vi "scan_waveform_yMirrored.vi"(6 "nlines":i32, 8 "flyback":i32, 9 "xpixels":i32, 10 "maxV":dbl, 11 "minV":dbl) -> (2 "xy scan waveform":dbl[][](array[numeric]))   [LabVIEW 2010]
panel:
  out "x waveform":dbl[](graph)
  out "y waveform":dbl[](graph)
  out "ystepSize":dbl
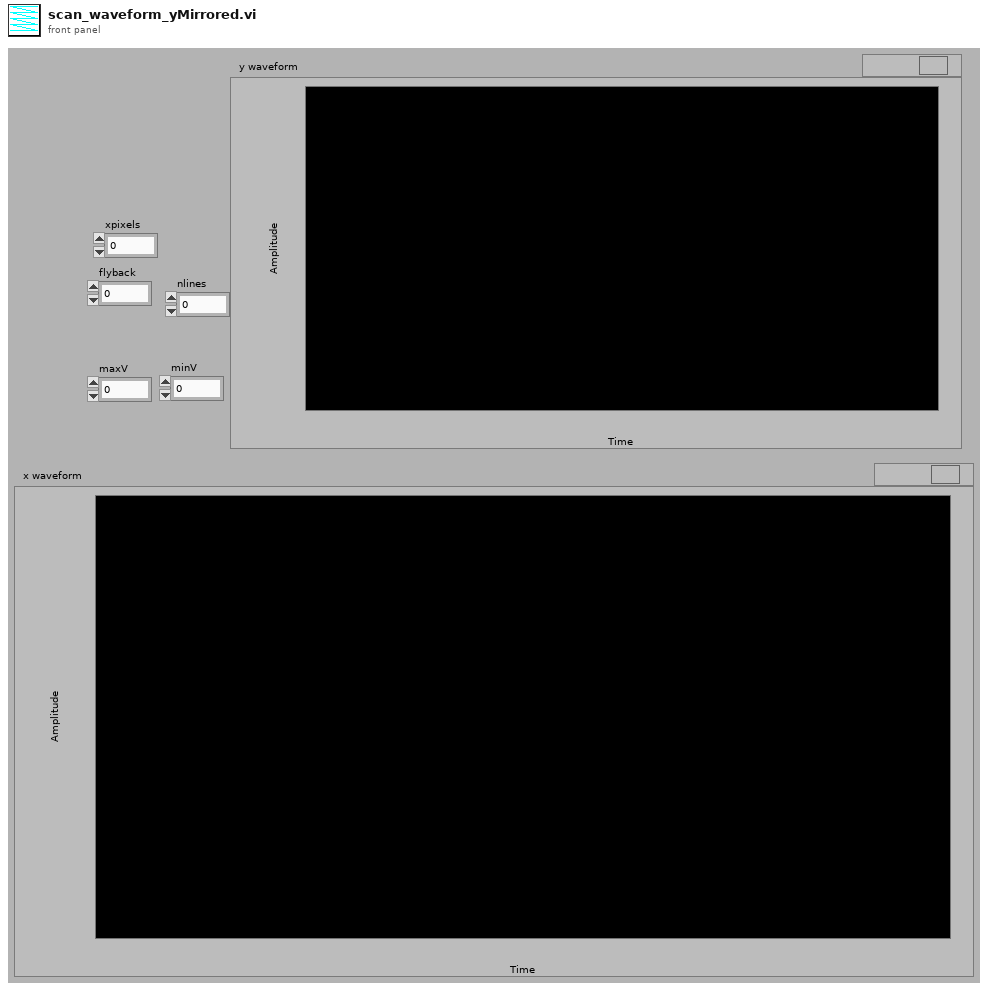
[diagram p1: front panel]
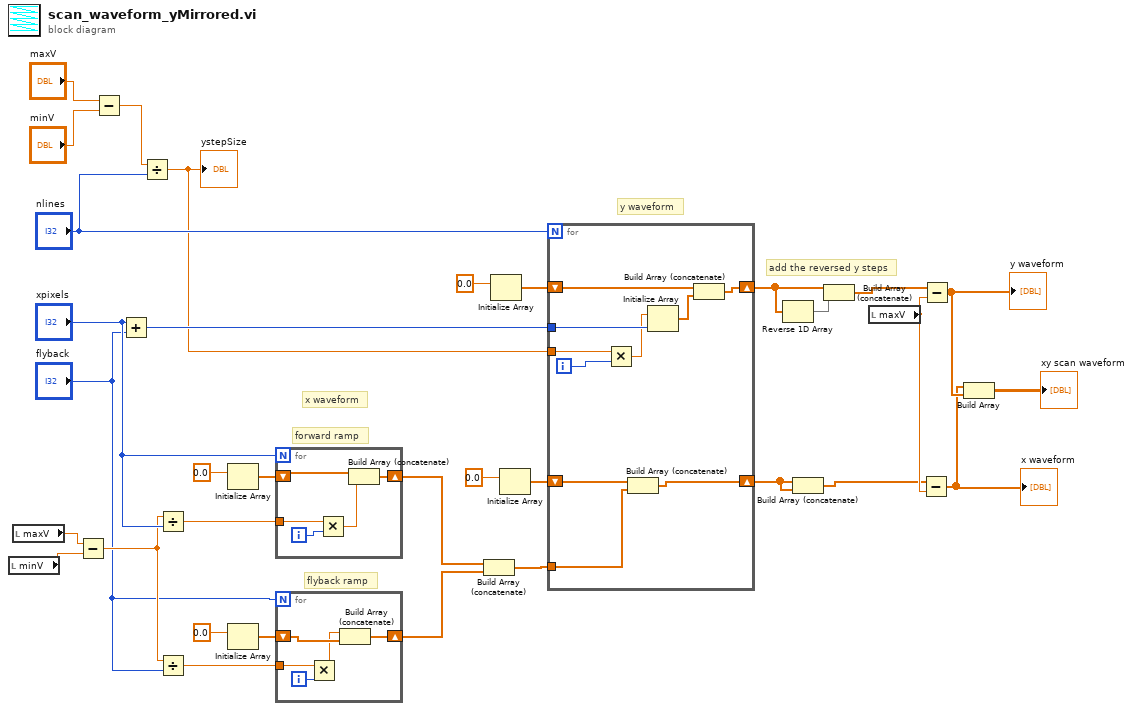
[diagram p0: block diagram]
diagram:
  # "add the reversed y steps"
  # "y waveform"
  # "x waveform"
  # "flyback ramp"
  # "forward ramp"
  n1 = local read "minV"() -> (w24:dbl)
  n2 = local read "maxV"() -> (w25:dbl)
  n3 = Subtract(x=w25, y=w24) -> (x-y=w13:dbl)
  n4 = Subtract(x="maxV", y="minV") -> (x-y=w7:dbl)
  n5 = Add(x="xpixels", y="flyback") -> (x+y=w28:i32)
  n6 = Divide(x=w7, y="nlines") -> (x/y=w10:dbl)
  "ystepSize" <- w10
  n7 = Divide(x=w13, y="xpixels") -> (x/y=w21:dbl)
  n8 = Divide(x=w13, y="flyback") -> (x/y=w20:dbl)
  n9 = Initialize Array(0.0 ("element")) -> (w26:dbl[])  [unwired: 1 out]
  n10 = Initialize Array(0.0 ("element")) -> (w23:dbl[])  [unwired: 1 out]
  n11 = for {
    N: "xpixels" -> [_]
    tunnel: w21 -> [w36]
    shift-right: [w34] -> w19
    shift-left: w26 -> [w38]
    i -> [w37]
    n12 = Multiply(x=w36, y=w37) -> (x*y=w35:dbl)
    n13 = Build Array (concatenate)(w38, w35) -> (w34:dbl[])
  }
  n14 = for {
    N: "flyback" -> [_]
    tunnel: w20 -> [w43]
    shift-right: [w41] -> w11
    shift-left: w23 -> [w40]
    i -> [w42]
    n15 = Multiply(x=w43, y=w42) -> (x*y=w39:dbl)
    n16 = Build Array (concatenate)(w39, w40) -> (w41:dbl[])
  }
  n17 = Build Array (concatenate)(w19, w11) -> (w16:dbl[])
  n18 = Initialize Array(0.0 ("element")) -> (w33:dbl[])  [unwired: 1 out]
  n19 = Initialize Array(0.0 ("element")) -> (w17:dbl[])  [unwired: 1 out]
  n20 = for {
    N: "nlines" -> [_]
    tunnel: w10 -> [w51]
    tunnel: w28 -> [w53]
    shift-right: [w47] -> w2
    shift-left: w33 -> [w48]
    shift-right: [w44] -> w1
    shift-left: w17 -> [w45]
    tunnel: w16 -> [w46]
    i -> [w52]
    n21 = Multiply(x=w51, y=w52) -> (x*y=w50:dbl)
    n22 = Build Array (concatenate)(w45, w46) -> (w44:dbl[])
    n23 = Initialize Array(w50, w53) -> (w49:dbl[])
    n24 = Build Array (concatenate)(w48, w49) -> (w47:dbl[])
  }
  n25 = Reverse 1D Array(array=w2) -> (reversed array=w3:dbl[])
  n26 = Build Array (concatenate)(w1, w1) -> (w9:dbl[])
  n27 = Build Array (concatenate)(w2, w3) -> (w8:dbl[])
  n28 = local read "maxV"() -> (w15:dbl)
  n29 = Subtract(x=w9, y=w15) -> (x-y=w5:dbl[])
  "x waveform" <- w5
  n30 = Subtract(x=w8, y=w15) -> (x-y=w6:dbl[])
  "y waveform" <- w6
  n31 = Build Array(w5, w6) -> (→"xy scan waveform":dbl[][])
